vi "XYindex 2 XYpos.vi"(0 "x_index":i32=44, 1 "y_index":i32=44, 2 "芯片角点坐标":T1={"x1(mm)"=1.0, "y1(mm)"=2.0, "x2(mm)"=1.0, "y2(mm)"=7.487, "x1 index"=0, "y1 index"=0, "x2 index"=0, "y2 index"=0, "Chip_POS"=[], "missing"=[]}) -> (3 "X当前坐标(mm)":dbl=1.0 format="%#.4f", 4 "Y当前坐标(mm)":dbl=7.4871486220076084 format="%#.4f", 5 "X当前坐标数":i32, 6 "Y当前坐标数":i32)   [LabVIEW 2013]
panel:
  in  "不再提示2":bool=TRUE
  in  "不再提示1":bool=TRUE
  out "y2_std":dbl
  out "x2_std":dbl
  out "y1_std":dbl
  out "x1_std":dbl
  out "dy1":dbl
  out "dy2":dbl
  out "dx2":dbl
  out "dx1":dbl
  out "dY":dbl
  out "dX":dbl
  out "theta":dbl
  out "y_std":dbl=3.88 format="%#.4f"
  out "x_std":dbl=3.88 format="%#.4f"
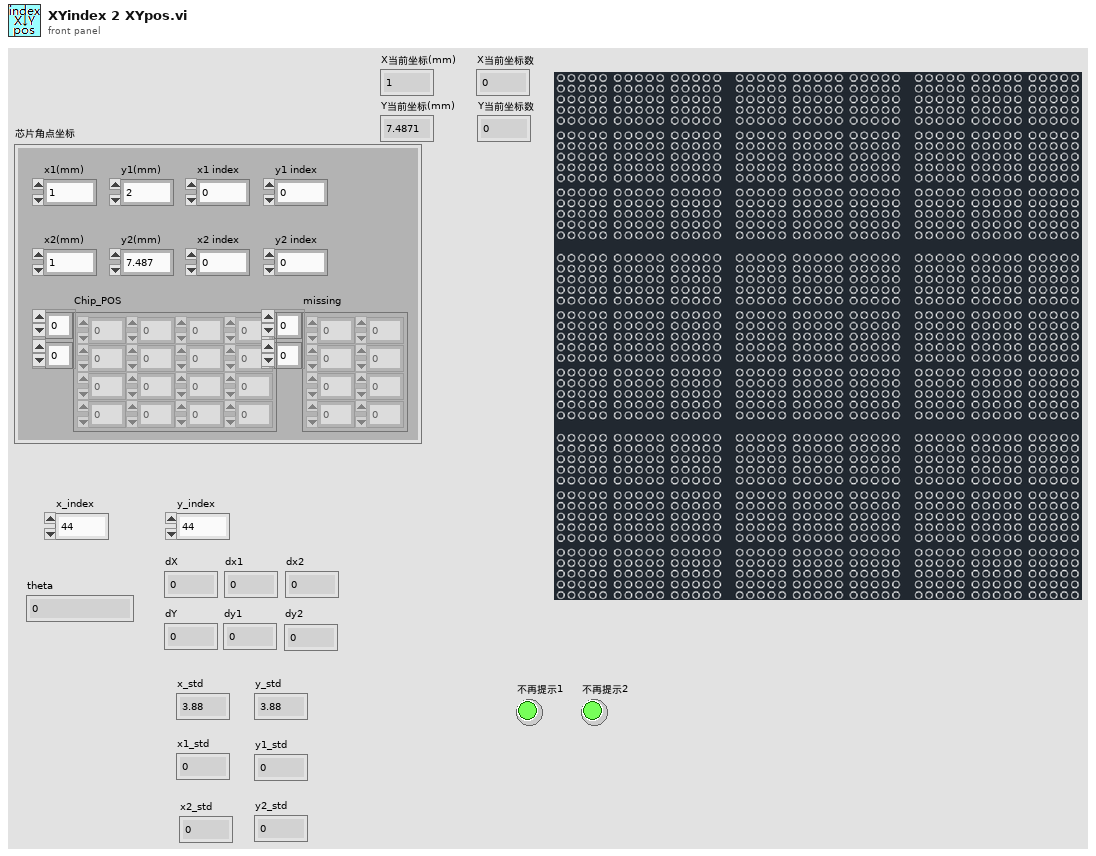
[diagram p1: front panel]
types:
  T1 = cluster{"x1(mm)":dbl, "y1(mm)":dbl, "x2(mm)":dbl, "y2(mm)":dbl, "x1 index":i32, "y1 index":i32, "x2 index":i32, "y2 index":i32, "Chip_POS":dbl[][], "missing":i32[][]}
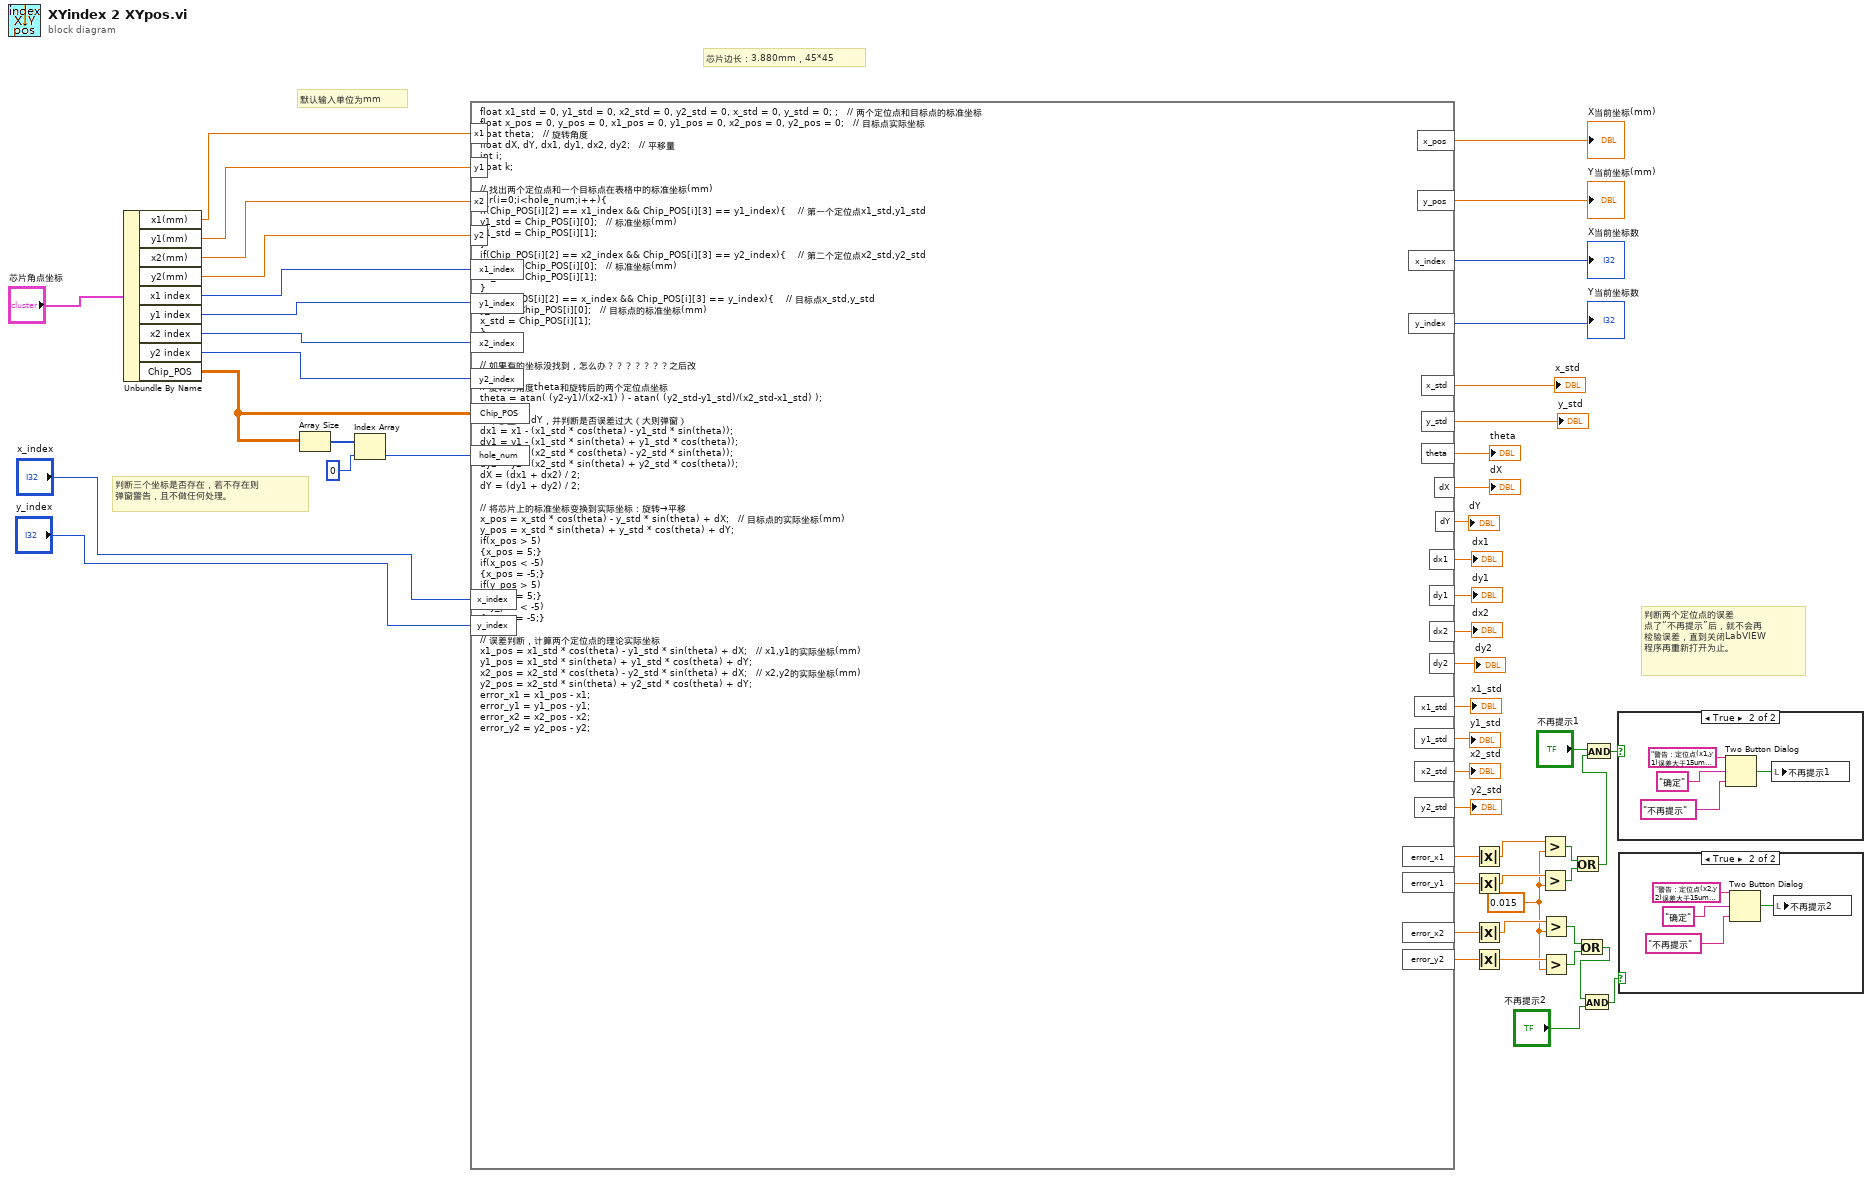
[diagram p0: block diagram]
diagram:
  w1 = 0.015 ("y")
  # "判断两个定位点的误差\n点了“不再提示”后，就不会再\n检验误差，直到关闭LabVIEW\n程序再重新打开为止。"
  # "判断三个坐标是否存在，若不存在则\n弹窗警告，且不做任何处理。"
  # "默认输入单位为mm"
  # "芯片边长：3.880mm，45*45"
  n1 = Unbundle By Name("芯片角点坐标") -> ("x1(mm)"=w51:dbl, "y1(mm)"=w50:dbl, "x2(mm)"=w49:dbl, "y2(mm)"=w48:dbl, "x1 index"=w46:i32, "y1 index"=w45:i32, "x2 index"=w44:i32, "y2 index"=w43:i32, "Chip_POS"=w47:dbl[][])
  n2 = Array Size(array=w47) -> (size(s)=w41:i32[])
  n3 = Index Array(array=w41, index=0 ("索引")) -> (element=w40:i32)
  n4 = formula code="float x1_std = 0, y1_std = 0, x2_std = 0, y2_std = 0, x_std = 0, y_std = 0; ;   // 两个定位点和目标点的标准坐标\nfloat x_pos = 0, y_pos = 0, x1_pos = 0, y1_pos = 0, x2_pos = 0, y2_pos = 0;   // 目标点实际坐标\nfloat theta;   // 旋转角度\nfloat dX, dY, dx1, dy1, dx2, dy2;   // 平移量\nint i;\nfloat k;\n\n// 找出两个定位点和一个目标点在表格中的标准坐标(mm)\nfor(i=0;i<hole_num;i++){\nif(Chip_POS[i][2] == x1_index && Chip_POS[i][3] == y1_index){    // 第一个定位点x1_std,y1_std\ny1_std = Chip_POS[i][0];   // 标准坐标(mm)\nx1_std = Chip_POS[i][1];\n}\nif(Chip_POS[i][2] == x2_index && Chip_POS[i][3] == y2_index){    // 第二个定位点x2_std,y2_std\ny2_std = Chip_POS[i][0];   // 标准坐标(mm)\nx2_std = Chip_POS[i][1];\n}\nif(Chip_POS[i][2] == x_index && Chip_POS[i][3] == y_index){    // 目标点x_std,y_std\ny_std = Chip_POS[i][0];   // 目标点的标准坐标(mm)\nx_std = Chip_POS[i][1];\n}\n}\n\n// 如果有的坐标没找到，怎么办？？？？？？？之后改\n\n// 旋转的角度theta和旋转后的两个定位点坐标\ntheta = atan( (y2-y1)/(x2-x1) ) - atan( (y2_std-y1_std)/(x2_std-x1_std) );\n\n// 平移量dX,dY，并判断是否误差过大（大则弹窗）\ndx1 = x1 - (x1_std * cos(theta) - y1_std * sin(theta));\ndy1 = y1 - (x1_std * sin(theta) + y1_std * cos(theta));\ndx2 = x2 - (x2_std * cos(theta) - y2_std * sin(theta));\ndy2 = y2 - (x2_std * sin(theta) + y2_std * cos(theta));\ndX = (dx1 + dx2) / 2;\ndY = (dy1 + dy2) / 2;\n\n// 将芯片上的标准坐标变换到实际坐标：旋转→平移\nx_pos = x_std * cos(theta) - y_std * sin(theta) + dX;   // 目标点的实际坐标(mm)\ny_pos = x_std * sin(theta) + y_std * cos(theta) + dY;\nif(x_pos > 5)\n{x_pos = 5;}\nif(x_pos < -5)\n{x_pos = -5;}\nif(y_pos > 5)\n{y_pos = 5;}\nif(y_pos < -5)\n{y_pos = -5;}\n\n// 误差判断，计算两个定位点的理论实际坐标\nx1_pos = x1_std * cos(theta) - y1_std * sin(theta) + dX;   // x1,y1的实际坐标(mm)\ny1_pos = x1_std * sin(theta) + y1_std * cos(theta) + dY;\nx2_pos = x2_std * cos(theta) - y2_std * sin(theta) + dX;   // x2,y2的实际坐标(mm)\ny2_pos = x2_std * sin(theta) + y2_std * cos(theta) + dY;\nerror_x1 = x1_pos - x1;\nerror_y1 = y1_pos - y1;\nerror_x2 = x2_pos - x2;\nerror_y2 = y2_pos - y2;"("x1"=w51, "y1"=w50, "x2"=w49, "y2"=w48, "x_index"="x_index", "y_index"="y_index", "Chip_POS"=w47, "hole_num"=w40, "x1_index"=w46, "y1_index"=w45, "x2_index"=w44, "y2_index"=w43) -> ("x_pos"=→"X当前坐标(mm)":dbl, "y_pos"=→"Y当前坐标(mm)":dbl, "x_std"=→"x_std":dbl, "y_std"=→"y_std":dbl, "theta"=→"theta":dbl, "dX"=→"dX":dbl, "dY"=→"dY":dbl, "dy1"=→"dy1":dbl, "dx1"=→"dx1":dbl, "dx2"=→"dx2":dbl, "dy2"=→"dy2":dbl, "x1_std"=→"x1_std":dbl, "y1_std"=→"y1_std":dbl, "x2_std"=→"x2_std":dbl, "y2_std"=→"y2_std":dbl, "error_x1"=w19:dbl, "x_index"=→"X当前坐标数":i32, "y_index"=→"Y当前坐标数":i32, "error_y1"=w18:dbl, "error_x2"=w16:dbl, "error_y2"=w17:dbl)
  n5 = Absolute Value(x=w19) -> (abs(x)=w15:dbl)
  n6 = Absolute Value(x=w18) -> (abs(x)=w14:dbl)
  n7 = Absolute Value(x=w16) -> (abs(x)=w13:dbl)
  n8 = Absolute Value(x=w17) -> (abs(x)=w12:dbl)
  n9 = Greater?(x=w15, y=w1) -> (0:w11:bool)
  n10 = Greater?(x=w14, y=w1) -> (0:w10:bool)
  n11 = Greater?(x=w13, y=w1) -> (0:w9:bool)
  n12 = Greater?(x=w12, y=w1) -> (0:w8:bool)
  n13 = Or(x=w11, y=w10) -> (x .or. y?=w6:bool)
  n14 = Or(x=w9, y=w8) -> (x .or. y?=w4:bool)
  n15 = And(x=w4, y="不再提示2") -> (x .and. y?=w3:bool)
  n16 = And(x="不再提示1", y=w6) -> (x .and. y?=w2:bool)
  n17 = case shown="True" w2 {
    frame False {
    }
    frame True {
      n18 = Two Button Dialog(message="警告：定位点(x1,y1)误差大于15um，可考虑重新定位或更换定位点。" ("消息"), 1:"不再提示" ("F按钮名称（“取消”）"), 2:"确定" ("按钮名称（“确定”）")) -> (T button?=w52:bool)
      n19 = local write "不再提示1"(w52) -> ()
    }
  }
  n20 = case shown="True" w3 {
    frame False {
    }
    frame True {
      n21 = Two Button Dialog(message="警告：定位点(x2,y2)误差大于15um，可考虑重新定位或更换定位点。" ("消息"), 1:"不再提示" ("F按钮名称（“取消”）"), 2:"确定" ("按钮名称（“确定”）")) -> (T button?=w56:bool)
      n22 = local write "不再提示2"(w56) -> ()
    }
  }
